vi "PeriodicFilter-Append Filtered Status.vi"(6 "Filtered Status":string[](array[string]), 11 "String Cache in":string) -> (0 "Filtered Status String":string, 3 "String Cache out":string)   [LabVIEW 2017, in "Communicable State Machine.lvlib"]
uses:
  Communicable State Machine.lvlib
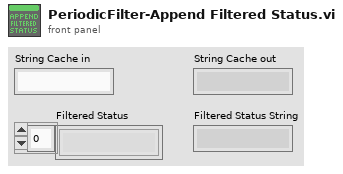
[diagram p1: front panel]
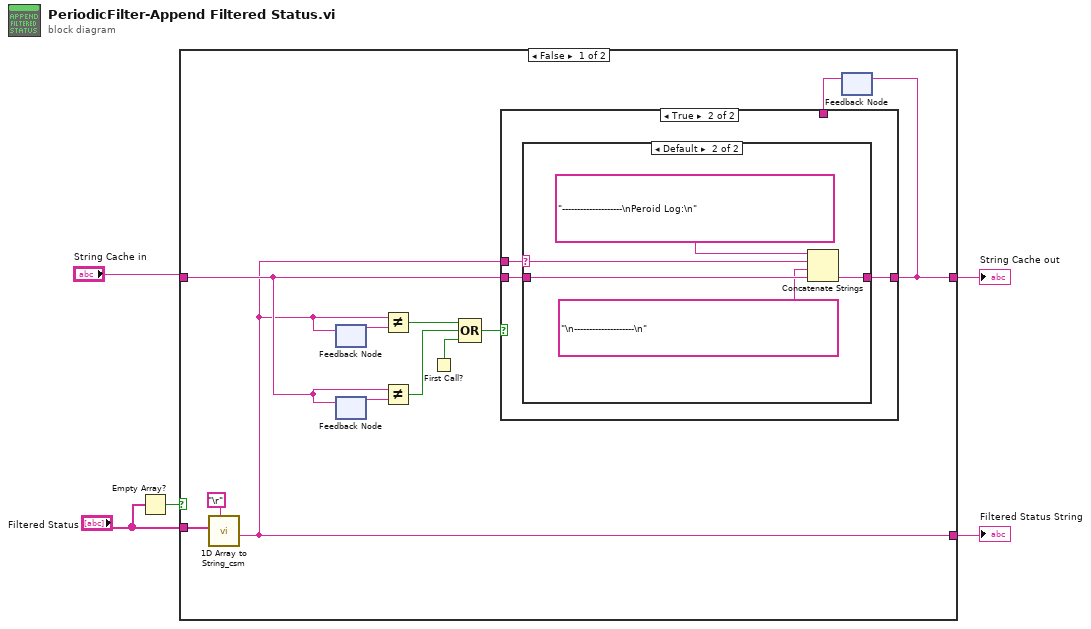
[diagram p0: block diagram]
diagram:
  n1 = Empty Array?(array="Filtered Status") -> (empty?=w5:bool)
  n2 = case shown="False" w5 {
    tunnel: [w8 _] -> w1
    tunnel: "String Cache in" -> [w10 w28]
    tunnel: [w16 w28] -> w3
    tunnel: "Filtered Status" -> [w14 _]
    frame False {
      n3 = call "1D Array to String_csm.vi"("delimiter (Tab)"="\r" ("Carriage Return Constant"), "Array of Strings"=w14) -> ("delimited string"=w8:string)  [unwired: 9 in]
      n4 = feedback #1() -> (w9:string)  [unwired: 1 in]
      n5 = feedback-in #1(w8) -> ()
      n6 = feedback #2() -> (w11:string)  [unwired: 1 in]
      n7 = feedback-in #2(w10) -> ()
      n8 = Not Equal?(x=w8, y=w9) -> (x != y?=w7:bool)
      n9 = Not Equal?(x=w10, y=w11) -> (x != y?=w12:bool)
      n10 = First Call?() -> (First Call?: T/F=w13:bool)
      n11 = Compound Arithmetic op=OR(w7, w12, w13) -> (w6:bool)
      n12 = feedback #3() -> (w15:string)  [unwired: 1 in]
      n13 = case shown="True" w6 {
        tunnel: [w18 w21] -> w16
        tunnel: w8 -> [_ w20]
        tunnel: w10 -> [_ w19]
        tunnel: w15 -> [w18 _]
        frame False {
        }
        frame True {
          n14 = case shown="Default" w20 {
            selector: w20 -> [_ w27]
            tunnel: w19 -> [w22 w26]
            tunnel: [w22 w25] -> w21
            frame "" {
            }
            frame Default {
              n15 = Concatenate Strings("--------------------\nPeroid Log:\n" ("string"), w27, "\n--------------------\n" ("string"), w26) -> (w25:string)
            }
          }
        }
      }
      n16 = feedback-in #3(w16) -> ()
    }
    frame True {
    }
  }
  "String Cache out" <- w3
  "Filtered Status String" <- w1
